vi "Update.vi"(8 "error in (no error)":errorcluster, 11 "Bouncer in":refnum<class "Bouncer.lvclass">) -> (0 "error out":errorcluster, 3 "Bouncer out":refnum<class "Bouncer.lvclass">)   [LabVIEW 2019, in "RT_Game.lvlib" / "Bouncer.lvclass"]
uses:
  Bouncer.lvclass
  C:/Users/FreshBob/Dropbox/VIs/myRIO_GameConsole/RT/RT_Game/Game/Game.lvclass
  PongBall/PongBall.lvclass
  C:/Users/FreshBob/Dropbox/VIs/myRIO_GameConsole/RT/RT_Game/GameObject/GameObject.lvclass
  Game/Game.lvclass/Game.ctl
  Bouncer.lvclass/Bouncer.ctl
  BounceTarget/BounceTarget.lvclass
  PongPanel/PongPanel.lvclass
  Game/Game.lvclass
  GameObject/GameObject.lvclass
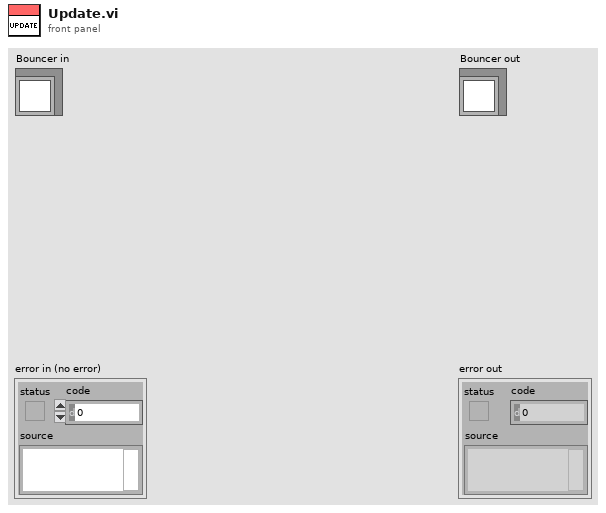
[diagram p1: front panel]
types:
  T1 = cluster{"Controls_1":cluster{"DirectionX":i8, "DirectionY":i8, "Button1":bool, "Button2":bool}, "Controls_2":cluster{"DirectionX":i8, "DirectionY":i8, "Button1":bool, "Button2":bool}, "SystemButton":bool}
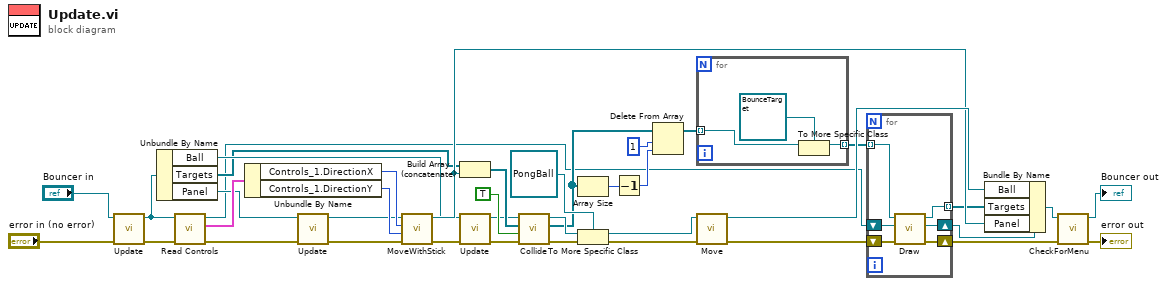
[diagram p0: block diagram]
diagram:
  n1 = call-parent "Update.vi"("error in (no error)"="error in (no error)", "Game in"="Bouncer in") -> ("error out"=w39:errorcluster, "Game out"=w23:refnum<class "Bouncer.lvclass">)  [unwired: 8 in]
  n2 = Unbundle By Name(w23) -> ("Ball"=w12:refnum<class "PongBall.lvclass">, "Targets"=w6:refnum<class "BounceTarget.lvclass">[], "Panel"=w8:refnum<class "PongPanel.lvclass">)
  n3 = call "Read Controls.vi"("error in (no error)"=w39, "Game in"=w23) -> ("error out"=w24:errorcluster, "Controls"=w22:T1, "Game out"=w4:refnum<class "Bouncer.lvclass">)  [unwired: 7 in]
  n4 = Unbundle By Name(w22) -> ("Controls_1.DirectionX"=w21:i8, "Controls_1.DirectionY"=w20:i8)
  n5 = call-dynamic "Update.vi"("error in (no error)"=w24, "GameObject in"=w8) -> ("error out"=w9:errorcluster, "GameObject out"=w7:refnum<class "PongPanel.lvclass">)  [unwired: 8 in]
  n6 = call "MoveWithStick.vi"("error in (no error)"=w9, "DirectionY"=w20, "DirectionX"=w21, "PongPanel in"=w7) -> ("error out"=w10:errorcluster, "PongPanel out"=w14:refnum<class "PongPanel.lvclass">)  [unwired: 6 in]
  n7 = Build Array (concatenate)(w6, w14) -> (w25:refnum<class "GameObject.lvclass">[])
  n8 = call-dynamic "Update.vi"("error in (no error)"=w10, "PongBall in"=w12) -> ("error out"=w13:errorcluster, "PongBall out"=w11:refnum<class "PongBall.lvclass">)  [unwired: 8 in]
  n9 = call "Collide.vi"("error in (no error)"=w13, "CollideAll?"=TRUE, "Colliders"=w25, "Object in"=w11) -> ("error out"=w36:errorcluster, "Colliders 2"=w19:refnum<class "GameObject.lvclass">[], "Object out"=w33:refnum<class "GameObject.lvclass">)  [unwired: 4 in, 1 out]
  n10 = Array Size(array=w19) -> (size(s)=w18:i32)
  n11 = To More Specific Class(target class=refnum<class "PongBall.lvclass"> refnum ("Ball"), reference=w33, error in=w36) -> (specific class reference=w30:refnum<class "PongBall.lvclass">, error out=w34:errorcluster)
  n12 = Decrement(x=w18) -> (x-1=w17:i32)
  n13 = Delete From Array(array=w19, length=1, index=w17) -> (array with subset deleted=w15:refnum<class "GameObject.lvclass">[])  [unwired: 1 out]
  n14 = for {
    tunnel: w15 -> [w41] mode=indexing
    tunnel: [w40] -> w2 mode=indexing
    n15 = To More Specific Class(target class=refnum<class "BounceTarget.lvclass"> refnum ("RT_Game.lvlib:BounceTarget.lvclass"), reference=w41) -> (specific class reference=w40:refnum<class "BounceTarget.lvclass">)  [unwired: 1 in, 1 out]
  }
  n16 = call "Move.vi"("error in (no error)"=w34, "PongBall in"=w30) -> ("error out"=w31:errorcluster, "PongBall out"=w28:refnum<class "PongBall.lvclass">)  [unwired: 8 in]
  n17 = for {
    shift-right: [w47] -> w5
    shift-left: w31 -> [w48]
    shift-right: [w45] -> w3
    shift-left: w4 -> [w46]
    tunnel: w2 -> [w44] mode=indexing
    tunnel: [w43] -> w1 mode=indexing
    n18 = call "Draw.vi"("error in (no error)"=w48, "RT_Game.lvlib:Game.lvclass"=w46, "BounceTarget in"=w44) -> ("error out"=w47:errorcluster, "RT_Game.lvlib:Game.lvclass 2"=w45:refnum<class "Bouncer.lvclass">, "BounceTarget out"=w43:refnum<class "BounceTarget.lvclass">)  [unwired: 6 in]
  }
  n19 = Bundle By Name(cluster=w3, "Ball"=w28, "Targets"=w1, "Panel"=w14) -> (w29:refnum<class "Bouncer.lvclass">)
  n20 = call "CheckForMenu.vi"("error in (no error)"=w5, "Snake in"=w29) -> ("error out"=→"error out":errorcluster, "Snake out"=→"Bouncer out":refnum<class "Bouncer.lvclass">)  [unwired: 8 in]
